vi "Oscillating_Body.vi"() -> ()   [LabVIEW 2015]
uses:
  <vilib>/Utility/error.llb/DialogType.ctl
  <vilib>/Analysis/baseanly.llb/Mean (DBL).vi
  <vilib>/Utility/file.llb/Read Delimited Spreadsheet (string).vi
  <vilib>/Analysis/NI_AALBase.lvlib
panel:
  in  "?":bool
  in  "Data Cluster":T1={"Reynolds No."="106666.66667", "Mach No."="0.028", "Red. Frequency - K"="0.2", "Mean AOA"="14", "Amp. AOA"="1", "Chord - mm"=160.0, "Span - mm"=305.0, "Run No."="01", "Pressure Coeff."=[], "Port Map"=[], "Nowind data"=[], "Pressure data (E)"=[], "AOA  (deg)"=[], "Uinf"=0.0, "Qinf"=0.0}
  in  "Run No.":string="01"
  in  "Amp. AOA":string="1"
  in  "Mean AOA":string="14"
  in  "Red. Frequency - K":string="0.2"
  in  "Mach No.":string="0.0871"
  in  "Reynolds No.":string="320000"
  out "Position of the Model":dbl[](graph)
  in  "Encoder Channel":T2={"Counter"="PXI1Slot4/ctr0", "A Input Terminal"="/PXI1Slot4/PFI8", "B Input Terminal"="/PXI1Slot4/PFI10", "Pulses Per Revolution"=2500, "Z Index Enable"=TRUE, "Z Index Terminal"="/PXI1Slot4/PFI9", "Rate (Hz)"=30000.0, "Duty Cycle"=0.9} {"Duty Cycle" format="%.6f"; "Rate (Hz)" format="%0.2f"}
  out "MIN AOA":dbl=-0.0
  out "MAX AOA":dbl=-0.0
  out "Uinf":dbl=20.13124742661755
  out "Qinf":dbl=239.1078838174274
  out "Exc":dbl=4.792962543727726 format="%.4f"
  in  "Span - mm":dbl=305.0
  in  "Chord - mm":dbl=160.0
  in  "OK Button":bool
  in  "stop":bool
  in  "Pressure Port Map File":path=path "C:/Users/KPoddar/Documents/Siva_Viknesh/Port_Map/N12_Port map.txt"
  in  "ESP DAQ Parameters":T3={"AI channels (ESP)"="PXI1Slot5/ai1:4, PXI1Slot5/ai0", "AI configuration"=10106, "DIO lines"="PXI1Slot5/port0/line0:7", "Counter Channel"="PXI1Slot5/ctr0", "Clock Source"="/PXI1Slot5/Ctr0InternalOutput", "Rate (Hz)"=30000.0, "Duty Cycle"=0.9} {"AI configuration" items=["default"=-1, "RSE"=10083, "NRSE"=10078, "Differential"=10106, "Pseudodifferential"=12529]; "Duty Cycle" format="%.6f"; "Rate (Hz)" format="%0.2f"}
  in  "Pressure Co-efficient File":path=path "C:/Users/KPoddar/Documents/Siva_Viknesh/ESP_Calibration/12_Jan_2019_Coeff"
  in  "Status":string="Acquiring WIND data"
  in  "start":bool
  out "Time Averaged - Cd":dbl(graph)=0.021300016641545187
  out "Time Averaged - Cn":dbl(graph)=-0.03572776492402335
  out "WAKE PROFILE":cluster{"y/c":dbl[], "u/U":dbl[]}[](graph)=[{"y/c"=[0.0, 0.125, 0.25, 0.375, 0.5, 0.625, 0.75, 0.875, 0.9375, 1.0, 1.0625, 1.125, 1.1875, 1.25, 1.3125, 1.375, 1.4375, 1.5, 1.5313, 1.5625, 1.5938, 1.625, 1.6563, 1.6875, 1.7188, 1.75, 1.7813, 1.8125, 1.8438, 1.875, 1.9063, 1.9375, 1.9688, 2.0, 2.0313, 2.0625, 2.0938, 2.125, 2.1563, 2.1875, 2.2188, 2.25, 2.2813, 2.3125, 2.375, 2.4375, 2.5, 2.5625, 2.625, 2.6875, 2.75, 2.8125, 2.875, 2.9375, 3.0625, 3.1875, 3.3125, 3.4375, 3.5625, 3.6875, 3.8125], "u/U"=[1.0009596796130957, 1.0006365708439775, 1.000458775077197, 1.0002151816823595, 0.9997285212941085, 0.9992218239397074, 0.9996159045344987, 0.9997997980670237, 0.9993085834876515, 0.9996161977909882, 0.9991442865487926, 0.9989225456627842, 0.9990589941645525, 0.9991516076620477, 0.9994968335049358, 0.9992479757372774, 0.9991270146766229, 0.9993130192283002, 0.9991894712210233, 0.9985573068874145, 0.9989133069802811, 0.9989284337914579, 0.9984919949101191, 0.9988670856422279, 0.998720478345178, 0.9988317138700255, 0.9987807809537579, 0.9993817728660642, 0.9991266204786825, 0.998687836529787, 0.9989096733798198, 0.9991314609754863, 0.9994357920312555, 0.9990554855328155, 0.9996339528050274, 0.9994616472312052, 0.998915988842227, 0.9990734865964254, 0.9994673752653088, 0.9919902882045858, 0.9477467514013836, 0.900572019686218, 0.9343035762242007, 0.9673359836539093, 0.9992770576762091, 0.9987392045631444, 0.9993232612300963, 0.9988661533943417, 0.9985982620956002, 0.9977815739815065, 0.9984383242595194, 0.997597623959294, 0.9991284364789002, 0.9988098962197963, 0.9984912543394804, 0.9989959032818851, 0.9986092133185214, 0.9996789602739807, 0.9992777829526237, 0.9998301775473059, 0.9989411932291912]}, {"y/c"=[2.5625, 2.5, 2.4375, 2.375, 2.3125, 2.2813, 2.25, 2.2188, 2.1875, 2.1563, 2.125, 2.0938, 2.0625, 2.0313], "u/U"=[0.9988661533943417, 0.9993232612300962, 0.9987392045631444, 0.999277057676209, 0.9673359836539093, 0.9343035762242007, 0.9005720196862179, 0.9477467514013836, 0.9919902882045857, 0.9994673752653088, 0.9990734865964253, 0.998915988842227, 0.9994616472312052, 0.9996339528050274]}]
  out "Cp Mean - Distribution":cluster{dbl[], dbl[]}[](graph)=[{[0.0, 0.0025, 0.0094, 0.0188, 0.0313, 0.0438, 0.0563, 0.0719, 0.0875, 0.1063, 0.125, 0.15, 0.175, 0.2125, 0.2563, 0.3125, 0.375, 0.4313, 0.4938, 0.55, 0.6125, 0.6813, 0.7438, 0.7969, 0.85, 0.9, 0.95, 1.0], [0.9895025094142684, 0.6723227895895574, 0.030036002629467956, -0.09402875024025721, -0.23779818113446574, -0.34455540345164654, -0.39132605168274986, -0.41420056762702084, -0.4342911435338544, -0.4413286241393345, -0.4378176575337153, -0.42907532072626553, -0.4108152467254266, -0.39188716231991094, -0.3664491451240933, -0.3311912285409058, -0.29730303730485924, -0.26694255938665684, -0.2328446524211739, -0.2039741062096574, -0.1696172409913368, -0.13486023803354916, -0.09125715168511339, -0.05034651463749375, -0.006449584802184226, 0.023613446884500216, 0.06775754964821469, 0.13681547205598854]}, {[0.0, 0.0031, 0.0113, 0.0225, 0.035, 0.05, 0.0688, 0.1, 0.1313, 0.175, 0.2313, 0.3063, 0.3938, 0.4938, 0.5938, 0.7, 0.8063, 0.9, 1.0], [0.9895025094142684, 0.5077403310445302, 0.0343588758716936, -0.15397968842982881, -0.25933078503216483, -0.3236102910091158, -0.39378422430067944, -0.4338455405586106, -0.4413534193685308, -0.4381014051616246, -0.42165505805841125, -0.38547160422512705, -0.340893512854035, -0.2850807623916184, -0.23051975129628735, -0.1728400176935098, -0.10194043390308628, -0.009577303812457928, 0.13681547205598854]}]
  in  "Scanner #":i32
  out "PRESSURE SIGNAL":dbl[][](graph)
  # "Pressure Measurement on Rotationally Oscillating Body - NACA 0012 Airfoil"
  # "ENCODER - SERVO MOTOR"
  # "MODEL PARAMETERS"
  # "Channel Parameters"
  # "Timing Parameters"
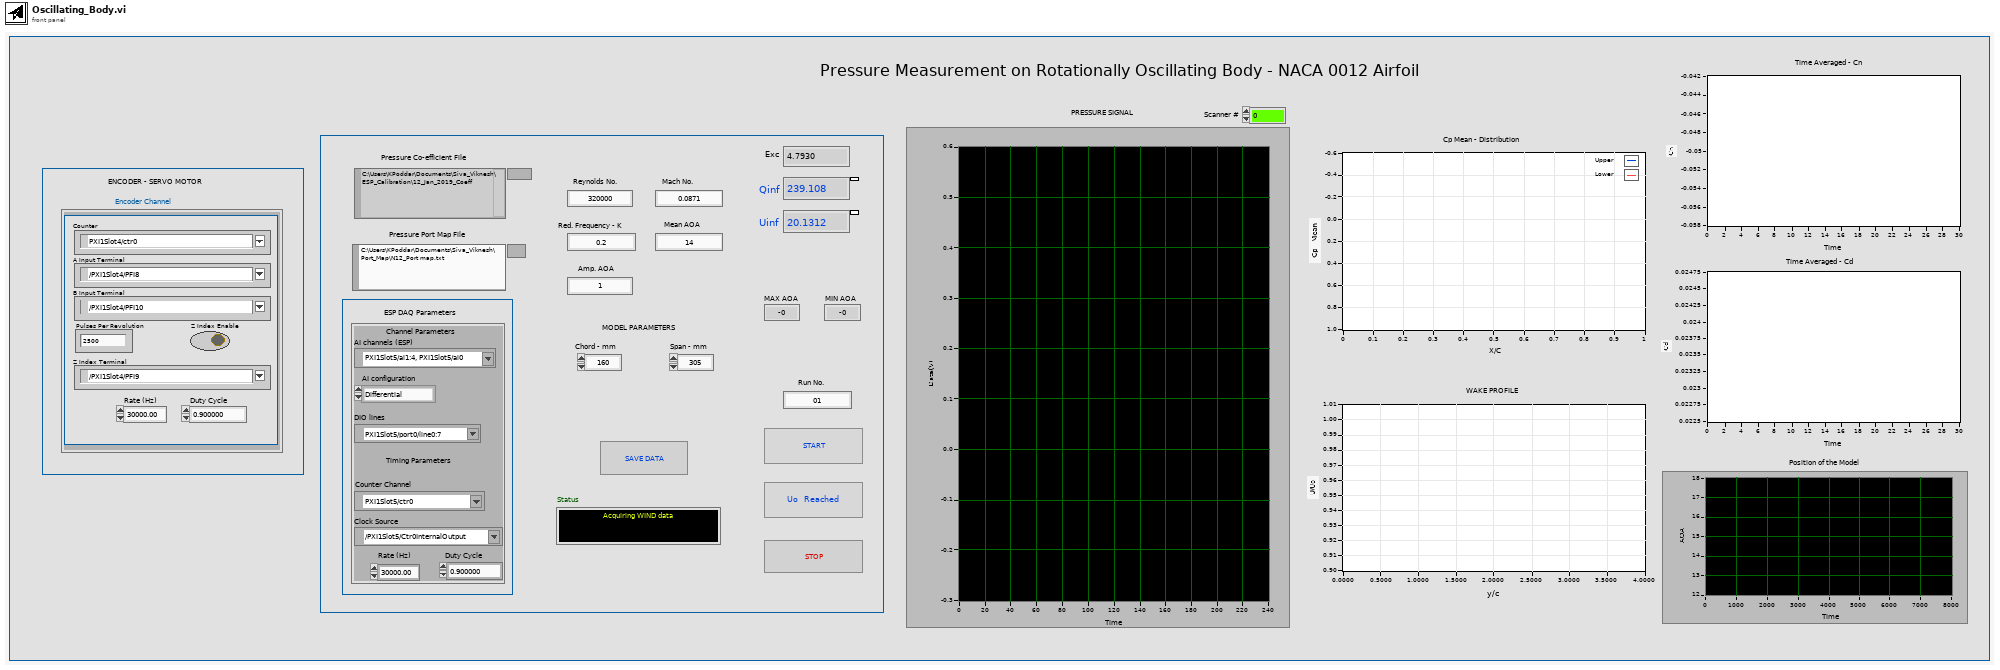
[diagram p1: front panel]
types:
  T1 = cluster{"Reynolds No.":string, "Mach No.":string, "Red. Frequency - K":string, "Mean AOA":string, "Amp. AOA":string, "Chord - mm":dbl, "Span - mm":dbl, "Run No.":string, "Pressure Coeff.":dbl[][][], "Port Map":dbl[][], "Nowind data":dbl[][], "Pressure data (E)":dbl[][][], "AOA  (deg)":dbl[], "Uinf":dbl, "Qinf":dbl}
  T2 = cluster{"Counter":tag, "A Input Terminal":tag, "B Input Terminal":tag, "Pulses Per Revolution":u32, "Z Index Enable":bool, "Z Index Terminal":tag, "Rate (Hz)":dbl, "Duty Cycle":dbl}
  T3 = cluster{"AI channels (ESP)":tag, "AI configuration":i32, "DIO lines":tag, "Counter Channel":tag, "Clock Source":tag, "Rate (Hz)":dbl, "Duty Cycle":dbl}
  T4 = typedef "DialogType.ctl" = u16
  T5 = enum16{"open", "replace", "create", "open or create", "replace or create", "replace or create with confirmation"}
  T6 = cluster{"Ucc (m/s)":dbl, "Cdp":dbl, "Cd ":dbl, "Cn":dbl, "Cmle":dbl, "Cmc/4":dbl, "Upp (m/s)":dbl, "AOA_Enc":dbl, "Cdc":dbl, "Qo (Pa)":dbl}
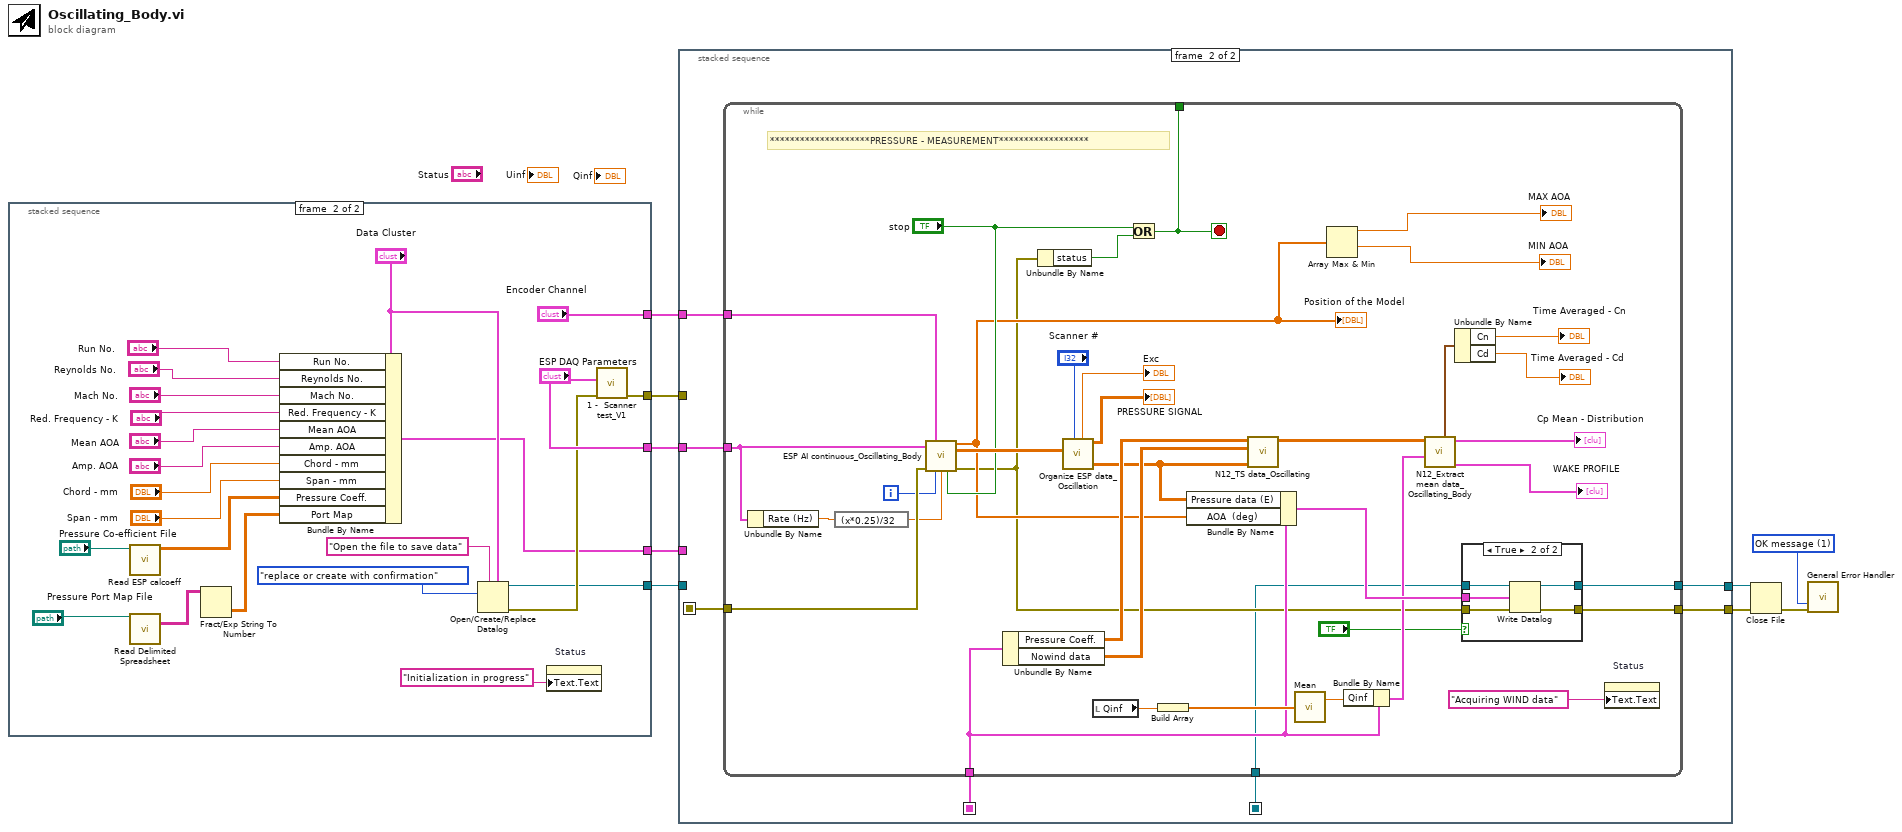
[diagram p0: block diagram]
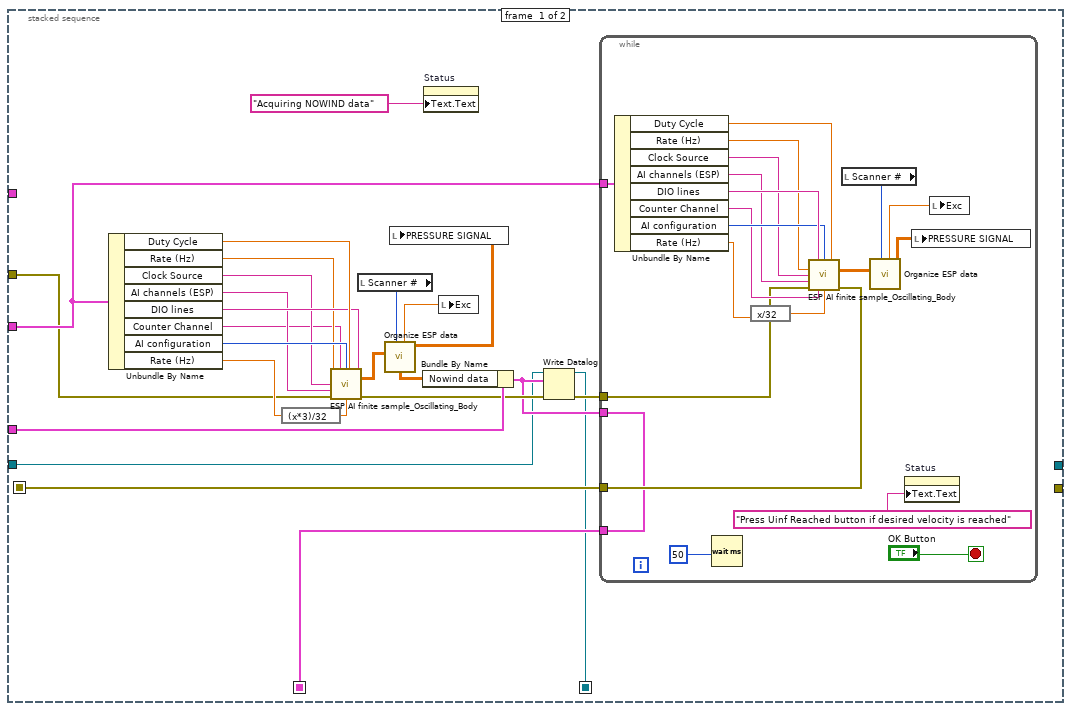
[diagram p2: hidden frame]
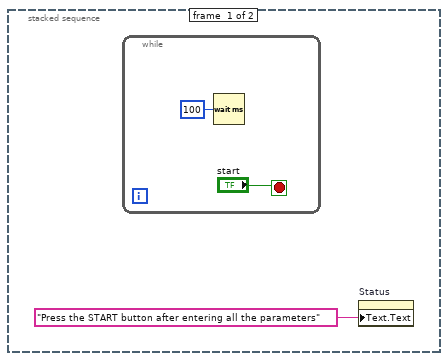
[diagram p4: hidden frame]
diagram:
  w7 = T4 1 items=["no dialog", "OK message", "continue or stop message", "OK message + warnings", "continue/stop + warnings"] ("type of dialog (OK msg:1)")
  n1 = stacked-sequence {
    tunnel: [_ w16] -> w2
    tunnel: [_ "ESP DAQ Parameters"] -> w9
    tunnel: [_ w15] -> w8
    tunnel: [_ "Encoder Channel"] -> w6
    tunnel: [_ w17] -> w1
    frame #0 {
      n2 = while {
        stop <- "start" stop-if-true
        n3 = Wait (ms)(milliseconds to wait=u32 100) -> ()  [unwired: 1 out]
      }
      n4 = property on="Status" class="Str"("Text.Text"="Press the START button after entering all the parameters") -> ()  [unwired: 2 in, 2 out]
    }
    frame #1 {
      n5 = call "Read ESP calcoeff.vi"("file path"="Pressure Co-efficient File") -> ("Scanner cal coefficients"=w22:dbl[][][])  [unwired: 7 in, 1 out]
      n6 = call-poly <vilib>:"Read Delimited Spreadsheet.vi"("file path (dialog if empty)"="Pressure Port Map File") -> ("all rows"=w21:string[][])  [unwired: 9 in, 5 out]
      n7 = Fract/Exp String To Number(string=w21) -> (number=w20:dbl[][])  [unwired: 4 out]
      n8 = Bundle By Name(cluster="Data Cluster", "Run No."="Run No.", "Reynolds No."="Reynolds No.", "Mach No."="Mach No.", "Red. Frequency - K"="Red. Frequency - K", "Mean AOA"="Mean AOA", "Amp. AOA"="Amp. AOA", "Chord - mm"="Chord - mm", "Span - mm"="Span - mm", "Pressure Coeff."=w22, "Port Map"=w20) -> (w15:T1)
      n9 = Open/Create/Replace Datalog(5:"Data Cluster", 7:"Open the file to save data" ("prompt"), 10:T5."replace or create with confirmation" ("operation (0:open)")) -> (0:w18:errorcluster, 3:w17:refnum<k1>)  [unwired: 3 in, 1 out]
      n10 = property on="Status" class="Str"("Text.Text"="Initialization in progress") -> ()  [unwired: 2 in, 2 out]
      n11 = call "1 -  Scanner test_V1.vi"("error in"=w18, "DAQ Parameters"="ESP DAQ Parameters") -> ("error out"=w16:errorcluster)  [unwired: 9 in]
    }
  }
  n12 = stacked-sequence {
    seq-local: [w43 _] -> [_ w84]
    seq-local: [w41 _] -> [_ w83]
    seq-local: [w36 _] -> [_ w81]
    tunnel: w9 -> [w44 w87]
    tunnel: w8 -> [w56 _]
    tunnel: [_ w86] -> w5
    tunnel: [_ w85] -> w4
    tunnel: w6 -> [_ w82]
    tunnel: w2 -> [w42 _]
    tunnel: w1 -> [w37 _]
    frame #0 {
      n13 = Unbundle By Name(w44) -> ("Duty Cycle"=w51:dbl, "Rate (Hz)"=w48:dbl, "Clock Source"=w47:tag, "AI channels (ESP)"=w46:tag, "DIO lines"=w50:tag, "Counter Channel"=w45:tag, "AI configuration"=w49:i32, "Rate (Hz)"=w59:dbl)
      n14 = expression code="(x*3)/32"(w59) -> (w58:dbl)
      n15 = call "ESP AI finite sample_Oscillating_Body.vi"("duty cycle"=w51, "DIO lines"=w50, "input terminal configuration"=w49, "Rate (Hz)"=w48, "Clock Source"=w47, "AI channels"=w46, "error in"=w42, "Counter Channel"=w45, "Nsamples"=w58) -> ("Pressure data out"=w57:dbl[][], "error out"=w40:errorcluster)  [unwired: 5 in]
      n16 = local read "Scanner #"() -> (w52:i32)
      n17 = call "Organize ESP data.vi"("Scanner"=w52, "Data in"=w57) -> ("Normalized scanner data"=w55:dbl[][], "Raw data"=w53:dbl[][], "Exc"=w54:dbl)  [unwired: 5 in]
      n18 = local write "PRESSURE SIGNAL"(w53) -> ()
      n19 = Bundle By Name(cluster=w56, "Nowind data"=w55) -> (w38:T1)
      n20 = property on="Status" class="Str"("Text.Text"="Acquiring NOWIND data") -> ()  [unwired: 2 in, 2 out]
      n21 = local write "Exc"(w54) -> ()
      n22 = Write Datalog(4:w40, 6:w38, 7:w37) -> (0:w39:errorcluster, 3:w36:refnum<k1>)
      n23 = while {
        tunnel: w44 -> [w75]
        tunnel: w38 -> [w61]
        tunnel: w39 -> [w63]
        tunnel: [w62] -> w43
        tunnel: [w61] -> w41
        stop <- "OK Button" stop-if-true
        n24 = Unbundle By Name(w75) -> ("Duty Cycle"=w69:dbl, "Rate (Hz)"=w67:dbl, "Clock Source"=w66:tag, "AI channels (ESP)"=w65:tag, "DIO lines"=w70:tag, "Counter Channel"=w64:tag, "AI configuration"=w68:i32, "Rate (Hz)"=w76:dbl)
        n25 = Wait (ms)(milliseconds to wait=u32 50) -> ()  [unwired: 1 out]
        n26 = expression code="x/32"(w76) -> (w74:dbl)
        n27 = call "ESP AI finite sample_Oscillating_Body.vi"("duty cycle"=w69, "DIO lines"=w70, "input terminal configuration"=w68, "Rate (Hz)"=w67, "Clock Source"=w66, "AI channels"=w65, "error in"=w63, "Counter Channel"=w64, "Nsamples"=w74) -> ("Pressure data out"=w77:dbl[][], "error out"=w62:errorcluster)  [unwired: 5 in]
        n28 = local read "Scanner #"() -> (w80:i32)
        n29 = call "Organize ESP data.vi"("Scanner"=w80, "Data in"=w77) -> ("Raw data"=w79:dbl[][], "Exc"=w78:dbl)  [unwired: 5 in, 1 out]
        n30 = property on="Status" class="Str"("Text.Text"="Press Uinf Reached button if desired velocity is reached") -> ()  [unwired: 2 in, 2 out]
        n31 = local write "PRESSURE SIGNAL"(w79) -> ()
        n32 = local write "Exc"(w78) -> ()
      }
    }
    frame #1 {
      n33 = while {
        tunnel: w87 -> [w124]
        tunnel: [w104] -> w86
        tunnel: [w103] -> w85
        tunnel: w84 -> [w123]
        tunnel: w83 -> [w92]
        tunnel: w82 -> [w98]
        tunnel: [w90] -> _
        tunnel: w81 -> [w88]
        i -> [w105]
        stop <- w90 stop-if-true
        # "********************PRESSURE - MEASUREMENT******************"
        n34 = Unbundle By Name(w124) -> ("Rate (Hz)"=w106:dbl)
        n35 = expression code="(x*0.25)/32"(w106) -> (w115:dbl)
        n36 = call "ESP AI continuous_Oscillating_Body.vi"("ESP DAQ Parameters"=w124, "ENCODER CHANNEL"=w98, "error in"=w123, "iteration"=w105, "Samples to read\n at a time"=w115, "clear acquisition"="stop") -> ("Current Position"=w93:dbl[], "Pressure data (E)"=w116:dbl[][], "error out"=w89:errorcluster)  [unwired: 7 in]
        "Position of the Model" <- w93
        n37 = Unbundle By Name(w92) -> ("Pressure Coeff."=w112:dbl[][][], "Nowind data"=w99:dbl[][])
        n38 = Unbundle By Name(w89) -> ("status"=w114:bool)
        n39 = call "Organize ESP data_Oscillation.vi"("Scanner"="Scanner #", "Data in"=w116) -> ("ESP data (V/Vexc)"=w97:dbl[][][], "ESP data (V)"=→"PRESSURE SIGNAL":dbl[][], "Exc"=→"Exc":dbl)  [unwired: 5 in]
        n40 = local read "Qinf"() -> (w96:dbl)
        n41 = Or(x="stop", y=w114) -> (x .or. y?=w90:bool)
        n42 = Build Array(w96) -> (w95:dbl[])
        n43 = Bundle By Name(cluster=w92, "Pressure data (E)"=w97, "AOA  (deg)"=w93) -> (w102:T1)
        n44 = call "N12_TS data_Oscillating.vi"("Pressure Coeff."=w112, "Nowind data"=w99, "ESP: wind data"=w97) -> ("Mean data"=w101:dbl[][])  [unwired: 5 in, 1 out]
        n45 = call-poly <vilib>:"Mean.vi"("X"=w95) -> ("mean"=w94:dbl)  [unwired: 1 out]
        n46 = Array Max & Min(array=w93) -> (max value=→"MAX AOA":dbl, min value=→"MIN AOA":dbl)  [unwired: 2 out]
        n47 = Bundle By Name(cluster=w92, "Qinf"=w94) -> (w100:T1)
        n48 = call "N12_Extract mean data_Oscillating_Body.vi"("Data Cluster"=w100, "Mean data"=w101) -> ("Wake profile_all"=→"WAKE PROFILE":cluster{"y/c":dbl[], "u/U":dbl[]}[], "Main Cp_mean"=→"Cp Mean - Distribution":cluster{"XL/C":dbl[], "Cpl":dbl[]}[], "Airfoil characteristics"=w111:T6)  [unwired: 3 in, 2 out]
        n49 = Unbundle By Name(w111) -> ("Cn"=→"Time Averaged - Cn":dbl, "Cd"=→"Time Averaged - Cd":dbl)
        n50 = case shown="True" "?" {
          tunnel: [w126 w131] -> w104
          tunnel: [w125 w130] -> w103
          tunnel: w102 -> [_ w129]
          tunnel: w89 -> [w125 w128]
          tunnel: w88 -> [w126 w127]
          frame False {
          }
          frame True {
            n51 = Write Datalog(4:w128, 6:w129, 7:w127) -> (0:w130:errorcluster, 3:w131:refnum<k1>)
          }
        }
        n52 = property on="Status" class="Str"("Text.Text"="Acquiring WIND data") -> ()  [unwired: 2 in, 2 out]
      }
    }
  }
  n53 = Close File(refnum=w5, error in=w4) -> (error out=w3:errorcluster)  [unwired: 1 out]
  n54 = call <vilib>:"General Error Handler.vi"("type of dialog (OK msg:1)"=w7, "error in (no error)"=w3) -> ()  [unwired: 9 in, 5 out]
